vi "Sensor Data (Multiple Readings).vi"(6 "Reading Interval (100)":dbl=100.0, 7 "Sample Count (1)":i32=1, 8 "error in (no error)":errorcluster, 9 "Data Source (0:Kelvin)":u16(ring) items=["Kelvin", "Celsius", "Sensor Units"], 10 "Sensor Input (0:A)":u16(ring) items=["A", "B"], 11 "VISA resource name":refnum<visa-resource-name>) -> (0 "error out":errorcluster, 2 "Sensor Data":dbl[](array[numeric]) format="%.4f", 3 "VISA resource name out":refnum<visa-resource-name>)   [LabVIEW 2019, in "Lake Shore 325.lvlib"]
doc: "Reads and returns multiple sensor readings from the instrument. Control over interval between readings is also provided."
uses:
  Lake Shore 325.lvlib
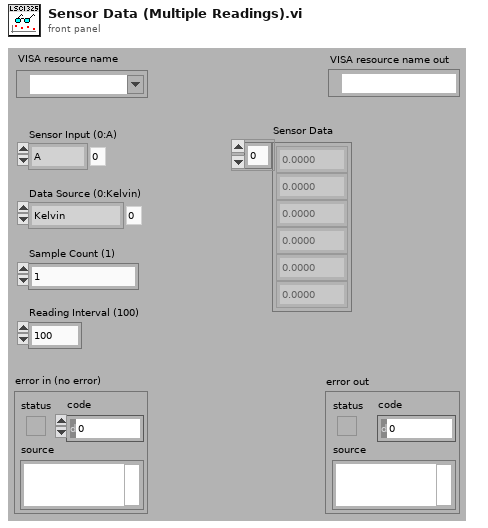
[diagram p1: front panel]
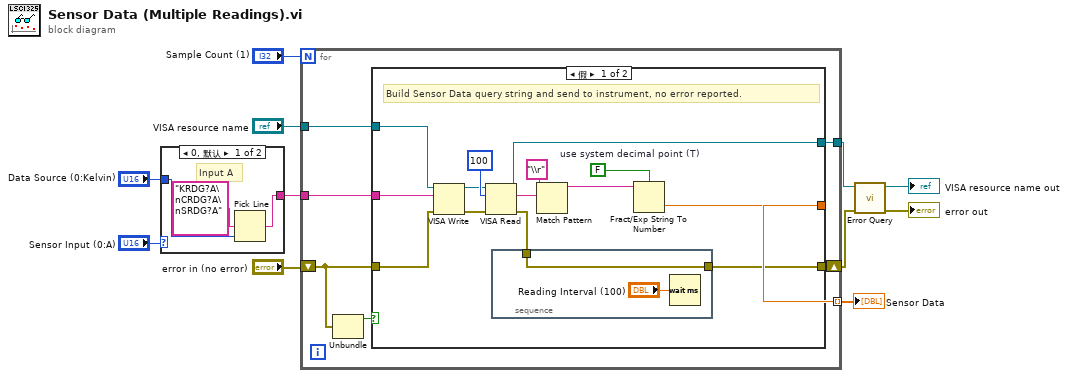
[diagram p0: block diagram]
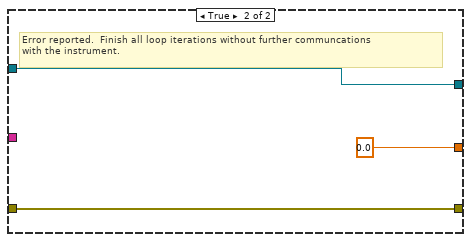
[diagram p2: hidden frame]
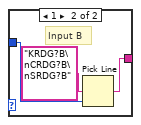
[diagram p3: hidden frame]
diagram:
  n1 = case shown="0, 默认" "Sensor Input (0:A)" {
    tunnel: "Data Source (0:Kelvin)" -> [w13 w15]
    tunnel: [w12 w16] -> w5
    frame 0, Default {
      # "Input A"
      n2 = Pick Line(multi-line string="KRDG?A\nCRDG?A\nSRDG?A", line index=w13) -> (output string=w12:string)  [unwired: 1 in]
    }
    frame 1 {
      # "Input B"
      n3 = Pick Line(multi-line string="KRDG?B\nCRDG?B\nSRDG?B", line index=w15) -> (output string=w16:string)  [unwired: 1 in]
    }
  }
  n4 = for {
    N: "Sample Count (1)" -> [_]
    tunnel: "VISA resource name" -> [w24]
    tunnel: [w23] -> w8
    tunnel: w5 -> [w22]
    tunnel: [w21] -> w3 mode=indexing
    shift-right: [w20] -> w1
    shift-left: "error in (no error)" -> [w19]
    n5 = Unbundle(w19) -> ("status"=w18:bool)  [unwired: 2 out]
    n6 = case shown="假" w18 {
      tunnel: w24 -> [w38 w43]
      tunnel: [w37 w43] -> w23
      tunnel: w22 -> [w29 _]
      tunnel: [w28 0.0] -> w21
      tunnel: w19 -> [w27 w42]
      tunnel: [w25 w42] -> w20
      frame False {
        w31 = FALSE  # use system decimal point (T)
        # "Build Sensor Data query string and send to instrument, no error reported."
        n7 = VISA Write(VISA resource name=w38, write buffer=w29, error in (no error)=w27) -> (VISA resource name out=w33:refnum<visa-resource-name>, error out=w32:errorcluster)  [unwired: 1 out]
        n8 = VISA Read(VISA resource name=w33, byte count=100, error in (no error)=w32) -> (VISA resource name out=w37:refnum<visa-resource-name>, read buffer=w35:string, error out=w26:errorcluster)  [unwired: 1 out]
        n9 = stacked-sequence {
          tunnel: w26 -> [w39]
          tunnel: [w39] -> w25
          frame #0 {
            n10 = Wait (ms)(milliseconds to wait="Reading Interval (100)") -> ()  [unwired: 1 out]
          }
        }
        n11 = Match Pattern(string=w35, regular expression="\\r") -> (before substring=w30:string)  [unwired: 1 in, 3 out]
        n12 = Fract/Exp String To Number(use system decimal point (T)=w31, string=w30) -> (number=w28:dbl)  [unwired: 2 in, 1 out]
      }
      frame True {
        # "Error reported.  Finish all loop iterations without further communcations\nwith the instrument."
      }
    }
  }
  "Sensor Data" <- w3
  n13 = call "Error Query.vi"("error in (no error)"=w1, "VISA resource name"=w8) -> ("error out"=→"error out":errorcluster, "VISA resource name out"=→"VISA resource name out":refnum<visa-resource-name>)  [unwired: 7 in, 1 out]
